vi "verifyThre.vi"(8 "error in (no error)":errorcluster, 11 "reference in":refnum<class "subject.lvclass">) -> (0 "error out":errorcluster, 1 "passThreshold":i32[](array[numeric]), 3 "reference out":refnum<class "subject.lvclass">)   [LabVIEW 2015, in "subject.lvclass"]
uses:
  subject.lvclass
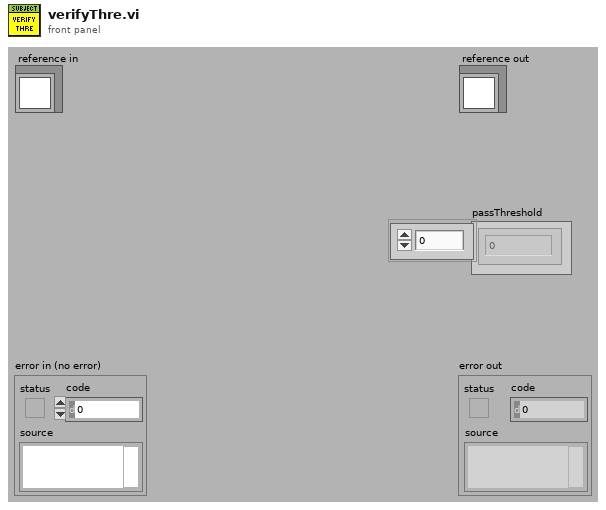
[diagram p1: front panel]
types:
  T1 = typedef "subject.lvclass/ObjectAttributesRef.ctl" = refnum<data-value>
  T2 = typedef "subject.lvclass/ObjectAttributes.ctl" = cluster{"MyAttribute":dbl, "data":cluster{"Ve_warm":dbl[], "time_warm":dbl[], "name":string, "phase":dbl[], "VCO2":dbl[], "VO2":dbl[], "PetCO2":dbl[], "RQ":dbl[], "HR":dbl[], "Ve_warm_inter":dbl[], "time_warm_inter":dbl[], "Ve_exer":dbl[], "time_exer":dbl[], "Ve_exer_inter":dbl[], "time_exer_inter":dbl[], "Ve":dbl[], "time":dbl[], "Ve_exer_inter_filtered":dbl[], "Ve_warm_inter_filtered":dbl[]}, "results_5l":cluster{"EOV":bool, "osci_amplitude":dbl[], "osci_width":dbl[], "peak_location":dbl[], "threshold":dbl, "width":i32}, "results_15percent":cluster{"EOV":bool, "osci_amplitude":dbl[], "osci_width":dbl[], "peak_location":dbl[], "threshold":dbl, "width":i32}, "supportData":cluster{"peaksAmplitude":dbl[], "iPeaksLocation":dbl[], "valesAmplitude":dbl[], "iValesLocation":dbl[], "threshold":dbl, "meanAmpl_warm":i32, "#_peaks":i32, "width":i32}, "results_user_selection":cluster{"EOV":bool, "osci_amplitude":dbl[], "osci_width":dbl[], "peak_location":dbl[], "threshold":dbl, "width":i32}, "results_warm_up":cluster{"EOV":bool, "osci_amplitude":dbl[], "osci_width":dbl[], "peak_location":dbl[], "threshold":dbl, "width":i32}}
  T3 = cluster{"peaksAmplitude":dbl[], "iPeaksLocation":dbl[], "valesAmplitude":dbl[], "iValesLocation":dbl[], "threshold":dbl, "meanAmpl_warm":i32, "#_peaks":i32, "width":i32}
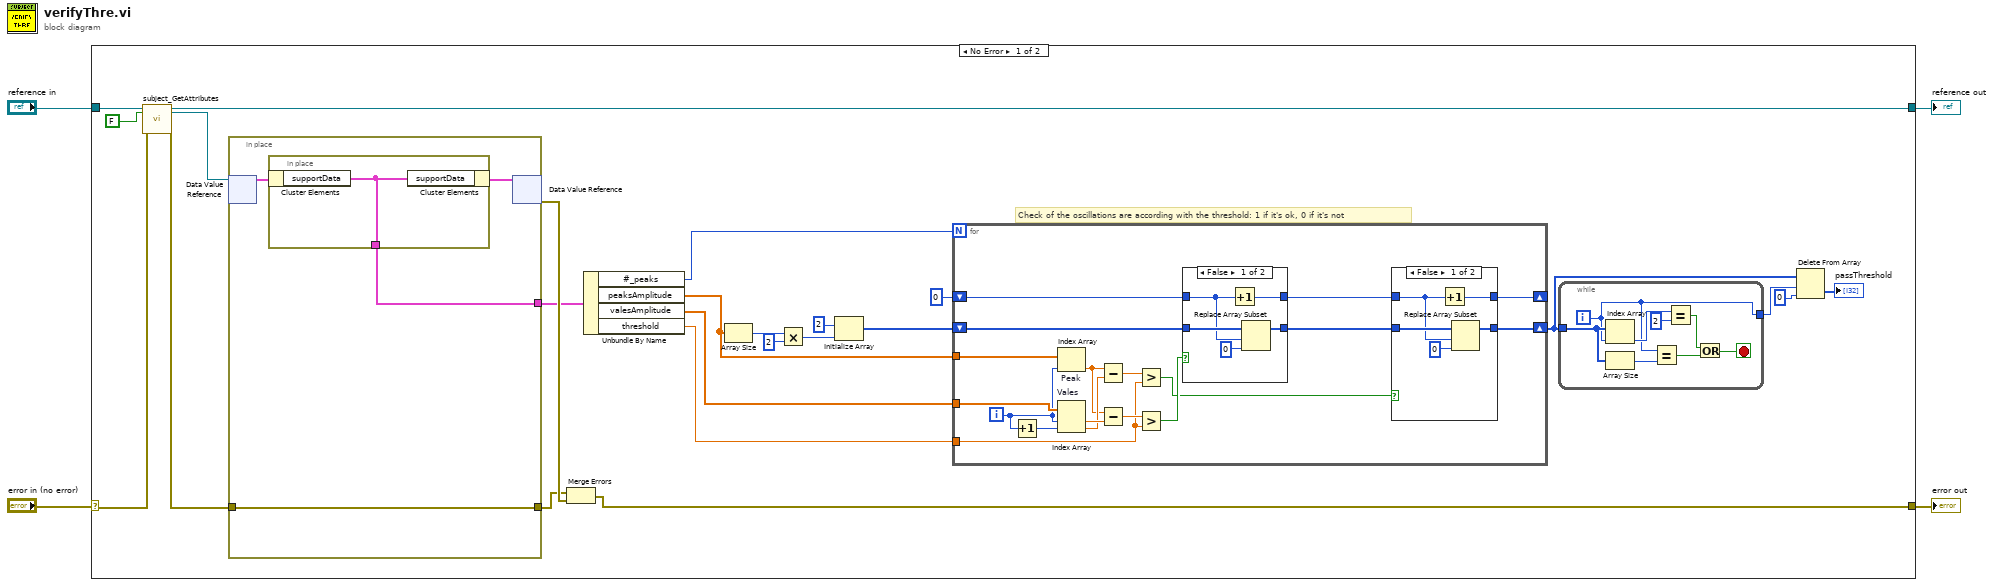
[diagram p0: block diagram]
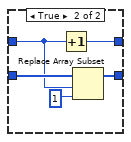
[diagram p2: hidden frame]
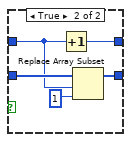
[diagram p3: hidden frame]
diagram:
  n1 = case shown="No Error" "error in (no error)" {
    selector: "error in (no error)" -> [w23 w81]
    tunnel: [w28 w81] -> w3
    tunnel: [w21 w80] -> w1
    tunnel: "reference in" -> [w25 w80]
    frame No Error {
      # "Check of the oscillations are according with the threshold: 1 if it's ok, 0 if it's not"
      n2 = call "subject_GetAttributes.vi"("reference in"=w25, "return data? (T)"=FALSE, "error in (no error)"=w23) -> ("reference out"=w21:refnum<class "subject.lvclass">, "attributes ref"=w20:T1, "error out"=w22:errorcluster)  [unwired: 13 in, 1 out]
      n3 = in-place {
        in-place-border: w22 -> [w76]
        in-place-border: [w76] -> w26
        in-place-border: [w75] -> w19
        n4 = in-place-dvr #1(w20) -> (w77:T2)  [unwired: 1 out]
        n5 = in-place {
          in-place-border: [w79] -> w75
          n6 = in-place-cluster #2(w77) -> ("supportData"=w79:T3)
          n7 = in-place-cluster #2("supportData"=w79) -> (w78:T2)
        }
        n8 = in-place-dvr #1(w78) -> (w27:errorcluster)  [unwired: 1 out]
      }
      n9 = Merge Errors(w26, w27) -> (w28:errorcluster)
      n10 = Unbundle By Name(w19) -> ("#_peaks"=w5:i32, "peaksAmplitude"=w6:dbl[], "valesAmplitude"=w7:dbl[], "threshold"=w8:dbl)
      n11 = Array Size(array=w6) -> (size(s)=w9:i32)
      n12 = Multiply(x=w9, y=2) -> (x*y=w12:i32)
      n13 = Initialize Array(2 ("element"), w12) -> (w13:i32[])
      n14 = for {
        N: w5 -> [_]
        tunnel: w6 -> [w54]
        tunnel: w7 -> [w47]
        tunnel: w8 -> [w51]
        shift-right: [w37] -> w15
        shift-left: w13 -> [w44]
        shift-right: [w39] -> _
        shift-left: 0 -> [w41]
        i -> [w43]
        n15 = Increment(x=w43) -> (x+1=w46:i32)
        n16 = Index Array "Peak"(array=w54, index=w43) -> (element=w48:dbl)
        n17 = Index Array "Vales"(array=w47, index #1=w43, index #2=w46) -> (element #1=w50:dbl, element #2=w49:dbl)
        n18 = Subtract(x=w48, y=w49) -> (x-y=w53:dbl)
        n19 = Subtract(x=w48, y=w50) -> (x-y=w52:dbl)
        n20 = Greater?(x=w53, y=w51) -> (0:w38:bool)
        n21 = Greater?(x=w52, y=w51) -> (0:w45:bool)
        n22 = case shown="False" w45 {
          tunnel: w44 -> [w69 w74]
          tunnel: [w67 w72] -> w42
          tunnel: w41 -> [w66 w70]
          tunnel: [w65 w71] -> w40
          frame False {
            n23 = Increment(x=w66) -> (x+1=w65:i32)
            n24 = Replace Array Subset(array=w69, new element=0 ("new element/subarray"), index=w66) -> (w67:i32[])
          }
          frame True {
            n25 = Increment(x=w70) -> (x+1=w71:i32)
            n26 = Replace Array Subset(array=w74, new element=1 ("new element/subarray"), index=w70) -> (w72:i32[])
          }
        }
        n27 = case shown="False" w38 {
          tunnel: w42 -> [w59 w63]
          tunnel: w40 -> [w56 w62]
          tunnel: [w58 w64] -> w39
          tunnel: [w57 w60] -> w37
          frame False {
            n28 = Increment(x=w56) -> (x+1=w58:i32)
            n29 = Replace Array Subset(array=w59, new element=0 ("new element/subarray"), index=w56) -> (w57:i32[])
          }
          frame True {
            n30 = Increment(x=w62) -> (x+1=w64:i32)
            n31 = Replace Array Subset(array=w63, new element=1 ("new element/subarray"), index=w62) -> (w60:i32[])
          }
        }
      }
      n32 = while {
        tunnel: w15 -> [w33]
        tunnel: [w29] -> w17
        i -> [w29]
        stop <- w30 stop-if-true
        n33 = Index Array(array=w33, index=w29) -> (element=w36:i32)
        n34 = Array Size(array=w33) -> (size(s)=w32:i32)
        n35 = Equal?(x=w29, y=w32) -> (x = y?=w31:bool)
        n36 = Equal?(x=w36, y=2) -> (x = y?=w34:bool)
        n37 = Or(x=w34, y=w31) -> (x .or. y?=w30:bool)
      }
      n38 = Delete From Array(array=w15, length=w17, index=0) -> (deleted portion=→"passThreshold":i32[])  [unwired: 1 out]
    }
    frame Error {
    }
  }
  "error out" <- w3
  "reference out" <- w1
